vi "Set Loss Units.vi"(8 "error in":errorcluster {"code" format="%.0x"}, 10 "Loss Unit":T1(ring), 11 "VISA resource name":refnum<visa-resource-name>) -> (0 "error out":errorcluster {"code" format="%.0x"}, 1 "Read string":string="UC= 9456.092   PF L= 658.76     NS V=0.10   V\r\n", 2 "Send string":string="UNITS 1;\nSHOW UN", 3 "VISA resource name out":refnum<visa-resource-name>)   [LabVIEW 2019, in "AH2500A.lvclass"]
uses:
  AH2500A.lvclass
panel:
  # "Set the lossunit"
  # "Default setting is 1"
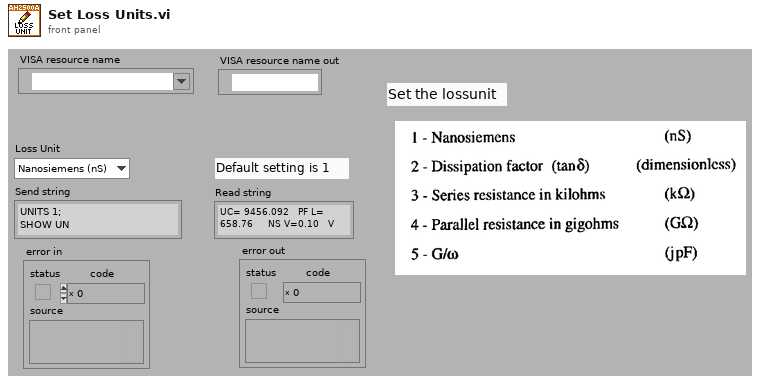
[diagram p1: front panel]
types:
  T1 = enum16{"Nanosiemens (nS)", "Dissipation (tan delta)", "Series R (kilohms)", "Parallel R (gigohms)", "G/omega (jpF)"}
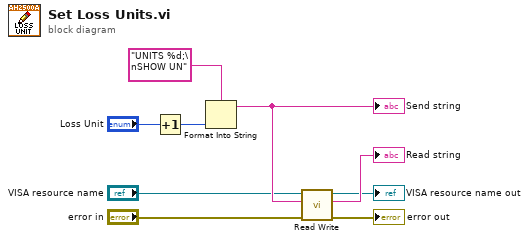
[diagram p0: block diagram]
diagram:
  n1 = Increment(x="Loss Unit") -> (x+1=w7:T1)
  n2 = Format Into String(format string="UNITS %d;\nSHOW UN", w7) -> (resulting string=w6:string)  [unwired: 2 in, 1 out]
  "Send string" <- w6
  n3 = call "Read Write.vi"("error in (no error)"="error in", "write buffer"=w6, "VISA Refnum in"="VISA resource name") -> ("error out"=→"error out":errorcluster, "read buffer"=→"Read string":string, "VISA Refnum out"=→"VISA resource name out":refnum<visa-resource-name>)  [unwired: 6 in]
